vi "Send Error Message.vi"(0 "Subject":string="Booth Error", 1 "Message":string="Hey Austin, \n\nSomething is wrong with the booth program", 3 "error in (no error)":errorcluster) -> (10 "error out":errorcluster)   [LabVIEW 2019]
uses:
  <vilib>/smtpClient/Set Message Text.vi
  <vilib>/smtpClient/LabVIEWSMTPClient.lvlib
panel:
  in  "TLS":bool=TRUE
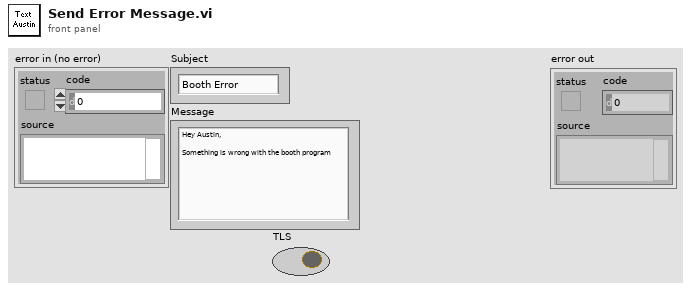
[diagram p1: front panel]
types:
  T1 = typedef "LabVIEWSMTPClient.lvlib/SmtpClientHandle.ctl" = refnum<k1>
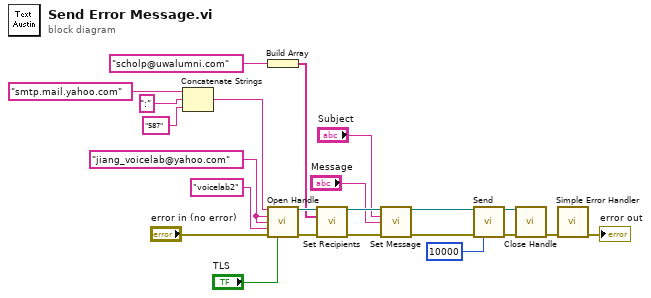
[diagram p0: block diagram]
diagram:
  w22 = "jiang_voicelab@yahoo.com" ("Email")
  n1 = Concatenate Strings("smtp.mail.yahoo.com" ("Outgoing Mail Server (SMTP)"), ":" ("string"), "587" ("Port")) -> (w7:string)
  n2 = Build Array("scholp@uwalumni.com" ("phone number")) -> (w11:string[])
  n3 = call <vilib>:"Open Handle.vi"("server address"=w7, "from"=w22, "username"=w22, "password"="voicelab2" ("Password"), "error in (no error)"="error in (no error)", "use TLS (false)"="TLS") -> ("handle out"=w23:T1, "error out"=w20:errorcluster)  [unwired: 8 in]
  n4 = call <vilib>:"Set Recipients.vi"("handle in"=w23, "to"=w11, "error in (no error)"=w20) -> ("handle out"=w19:T1, "error out"=w18:errorcluster)  [unwired: 11 in]
  n5 = call-poly <vilib>:"Set Message.vi"("handle in"=w19, "subject"="Subject", "plain text message"="Message", "error in (no error)"=w18) -> ("handle out"=w15:T1, "error out"=w14:errorcluster)  [unwired: 10 in]
  n6 = call <vilib>:"Send.vi"("handle in"=w15, "error in (no error)"=w14, "timeout in ms (10000)"=10000) -> ("handle out"=w13:T1, "error out"=w12:errorcluster)  [unwired: 10 in, 1 out]
  n7 = call <vilib>:"Close Handle.vi"("handle in"=w13, "error in (no error)"=w12) -> ("error out"=w4:errorcluster)  [unwired: 12 in, 1 out]
  n8 = call <vilib>:"Simple Error Handler.vi"("error in (no error)"=w4) -> ("error out"=→"error out":errorcluster)  [unwired: 4 in, 4 out]
